vi "Config to table.vi"(10 "engine configuration":refnum<class "engine configuration.lvclass">, 11 "tag select module configuration in":refnum<class "tag select module configuration.lvclass">) -> (3 "Array":string[][](array[string]))   [LabVIEW 2013]
uses:
  <vilib>/NI/Module Execution Interface/Engine Configuration/engine configuration.lvclass
  module/configuration/tag select module configuration.lvclass
  module/configuration/tag select module configuration.lvclass/tag select module configuration.ctl
  <vilib>/NI/Configuration Framework/serializable configuration/NISE_CEF_serializable configuration.lvclass/NISE_CEF_serializable configuration.ctl
  <vilib>/NI/Tag Bus/tag/tag descriptor.lvclass/tag descriptor.ctl
  module/configuration/Read tag select.vi
  <vilib>/Utility/LVClass/Get LV Class Name.vi
  <vilib>/NI/Configuration Framework/error generator/NISE_error generator.vi
  <vilib>/NI/Tag Bus/tag/tag descriptor.lvclass
  <vilib>/NI/Configuration Framework/serializable configuration/NISE_CEF_serializable configuration.lvclass
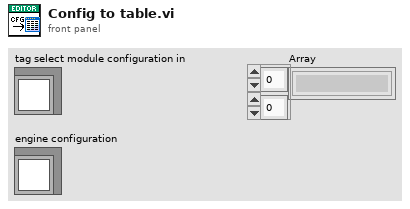
[diagram p1: front panel]
types:
  T1 = typedef "tag select module configuration.lvclass/tag select configuration.ctl" = cluster{"tag select name":string, "data type":T2, "output":refnum<class "TBM channel.lvclass">, "select":refnum<class "TBM channel.lvclass">, "input channels":refnum<class "TBM channel.lvclass">[]}
  T2 = typedef "tag bus.lvlib/tag descriptor.lvclass/Data Type.ctl" = enum16{"Double", "Single", "I64", "I32", "I16", "I8", "U64", "U32", "U16", "U8", "Boolean", "String", "Array of Double", "Array of Single", "Array of I64", "Array of I32", "Array of I16", "Array of I8", "Array of U64", "Array of U32", "Array of U16", "Array of U8", "Array of Boolean", "Array of String"}
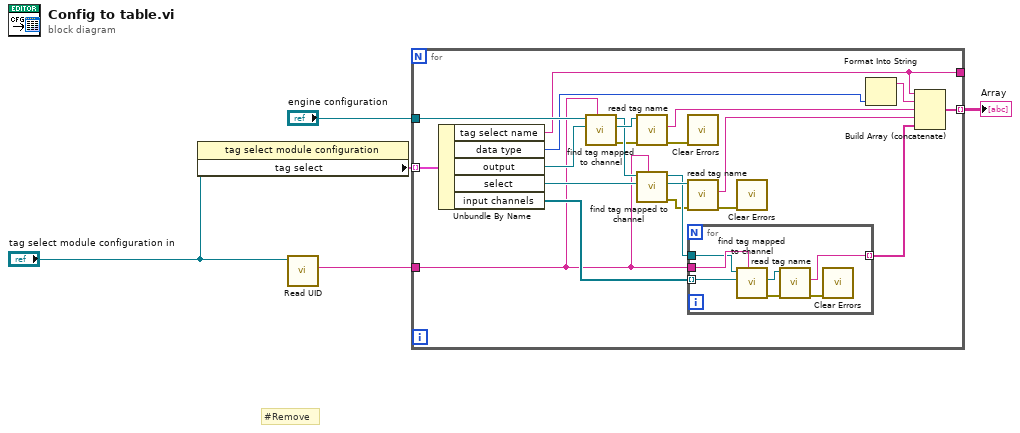
[diagram p0: block diagram]
diagram:
  # "#Remove"
  n1 = property class="tag select module configuration"(reference="tag select module configuration in") -> ("tag select"=w2:T1[])  [unwired: 1 in, 2 out]
  n2 = call <vilib>:"Read UID.vi"("configuration in"="tag select module configuration in") -> ("instance id"=w4:string)  [unwired: 8 in, 2 out]
  n3 = for {
    tunnel: w2 -> [w26] mode=indexing
    tunnel: [w17] -> _
    tunnel: "engine configuration" -> [w25]
    tunnel: w4 -> [w6]
    tunnel: [w13] -> w5 mode=indexing
    n4 = Unbundle By Name(w26) -> ("tag select name"=w17:string, "data type"=w16:T2, "output"=w22:refnum<class "TBM channel.lvclass">, "select"=w21:refnum<class "TBM channel.lvclass">, "input channels"=w23:refnum<class "TBM channel.lvclass">[])
    n5 = call <vilib>:"find tag mapped to channel.vi"("owner"=w6, "channel"=w22, "engine configuration in"=w25) -> ("error out"=w10:errorcluster, "tag"=w24:refnum<class "tag descriptor.lvclass">, "engine configuration out"=w11:refnum<class "engine configuration.lvclass">)  [unwired: 6 in]
    n6 = call <vilib>:"read tag name.vi"("error in"=w10, "system tag in"=w24) -> ("error out"=w7:errorcluster, "name"=w20:string)  [unwired: 7 in, 1 out]
    n7 = call <vilib>:"find tag mapped to channel.vi"("owner"=w6, "channel"=w21, "engine configuration in"=w11) -> ("error out"=w9:errorcluster, "tag"=w19:refnum<class "tag descriptor.lvclass">, "engine configuration out"=w12:refnum<class "engine configuration.lvclass">)  [unwired: 6 in]
    n8 = call <vilib>:"Clear Errors.vi"("error in (no error)"=w7) -> ()  [unwired: 6 in, 1 out]
    n9 = call <vilib>:"read tag name.vi"("error in"=w9, "system tag in"=w19) -> ("error out"=w8:errorcluster, "name"=w18:string)  [unwired: 7 in, 1 out]
    n10 = for {
      tunnel: w6 -> [w33]
      tunnel: w23 -> [w32] mode=indexing
      tunnel: [w30] -> w14 mode=indexing
      tunnel: w12 -> [w29]
      n11 = call <vilib>:"find tag mapped to channel.vi"("owner"=w33, "channel"=w32, "engine configuration in"=w29) -> ("error out"=w28:errorcluster, "tag"=w31:refnum<class "tag descriptor.lvclass">)  [unwired: 6 in, 1 out]
      n12 = call <vilib>:"read tag name.vi"("error in"=w28, "system tag in"=w31) -> ("error out"=w27:errorcluster, "name"=w30:string)  [unwired: 7 in, 1 out]
      n13 = call <vilib>:"Clear Errors.vi"("error in (no error)"=w27) -> ()  [unwired: 6 in, 1 out]
    }
    n14 = call <vilib>:"Clear Errors.vi"("error in (no error)"=w8) -> ()  [unwired: 6 in, 1 out]
    n15 = Format Into String(w16) -> (resulting string=w15:string)  [unwired: 3 in, 1 out]
    n16 = Build Array (concatenate)(w17, w15, w20, w18, w14) -> (w13:string[])
  }
  "Array" <- w5
